vi "WPI_SonarSRF04DigitalOpen.vi"(8 "error in (no error)":errorcluster, 9 "Echo DIO Channel":T1=enum."DIO 2", 11 "Ping DIO Channel":T1=enum."DIO 1") -> (0 "error out":errorcluster, 3 "UltrasonicDevRef":T2={"DevStatus"={"status"=FALSE, "code"=0, "source"=""}, "Ping Channel"=enum."Invalid", "Echo Channel"=enum."Invalid", "CntIndex"=enum."Invalid"})   [LabVIEW 2017]
doc: "Creates a reference to the ultrasonic sensor you specify. You must open a reference before using any other VIs on this palette.\n\nThis software is licensed. Open the labview\\readme\\WPI Robotics Library Open Source License.txt file for more information."
uses:
  <vilib>/Rock Robotics/WPI/Ultrasonic/WPI_UltrasonicDeviceRef.ctl
  <vilib>/Rock Robotics/SystemInterfaces/DIO/FPGA_DIOChannel.ctl
  <vilib>/Rock Robotics/SystemInterfaces/Counter/FPGA_CounterCtrSystemIndex.ctl
  <vilib>/robotics/Simulator/Engine/ctl/DeviceID.ctl
  <vilib>/Rock Robotics/WPI/Counter/WPI_CounterDigitalInputToDigitalSource.vi
  <vilib>/Rock Robotics/WPI/Counter/WPI_CounterOpen Semi Period Mode.vi
  <instrlib>/Devantech SRF05/HAIOL/Simulator/Devantech SRF05 Simulator.lvclass
  <vilib>/robotics/Simulator/NI_Robotics_Simulator.lvlib
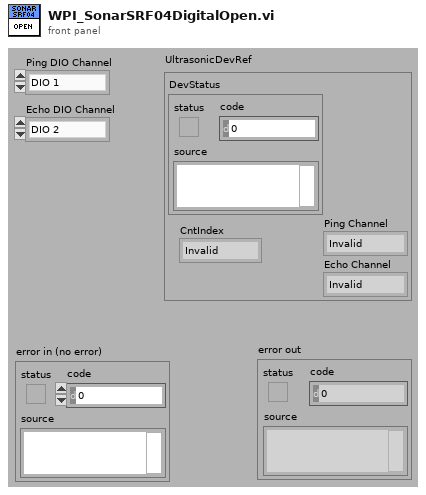
[diagram p1: front panel]
types:
  T1 = typedef "FPGA_DIOChannel.ctl" = enum8{"DIO 0", "DIO 1", "DIO 2", "DIO 3", "DIO 4", "DIO 5", "DIO 6", "DIO 7", "DIO 8", "DIO 9", "DIO MXP 0", "DIO MXP 1", "DIO MXP 2", "DIO MXP 3", "DIO MXP 4", "DIO MXP 5", "DIO MXP 6", "DIO MXP 7", "DIO MXP 8", "DIO MXP 9", "DIO MXP 10", "DIO MXP 11", "DIO MXP 12", "DIO MXP 13", "DIO MXP 14", "DIO MXP 15", "SPI Port CS1", "SPI Port CS2", "SPI Port CS3", "SPI Port MISO", "SPI Port MOSI", "Invalid"}
  T2 = typedef "WPI_UltrasonicDeviceRef.ctl" = cluster{"DevStatus":errorcluster, "Ping Channel":T1, "Echo Channel":T1, "CntIndex":T3}
  T3 = typedef "FPGA_CounterCtrSystemIndex.ctl" = enum8{"Ctr 0", "Ctr 1", "Ctr 2", "Ctr 3", "Ctr 4", "Ctr 5", "Ctr 6", "Ctr 7", "Invalid"}
  T4 = typedef "NI_Robotics_Simulator.lvlib/DeviceID.ctl" = cluster{"robot ID":string, "sensor/actuator ID":string}
  T5 = typedef "WPI_DigitalInputDevRef.ctl" = cluster{"DevStatus":errorcluster, "DIO Channel":T1}
  T6 = typedef "FPGA_CounterEncoderSourceConvertionLVSourceType.ctl" = cluster{"DevStatus":errorcluster, "AnalogTriggerMode?":bool, "DigitalMode":cluster{"DIO Channel":T7}, "AnalogTriggerMode":cluster{"AnalogTriggerIndex":T8, "OutputType":T9}}
  T7 = typedef "FPGA_DIODigitalSourceChannel.ctl" = enum8{"DIO 0", "DIO 1", "DIO 2", "DIO 3", "DIO 4", "DIO 5", "DIO 6", "DIO 7", "DIO 8", "DIO 9", "DIO MXP 0", "DIO MXP 1", "DIO MXP 2", "DIO MXP 3", "DIO MXP 4", "DIO MXP 5", "DIO MXP 6", "DIO MXP 7", "DIO MXP 8", "DIO MXP 9", "DIO MXP 10", "DIO MXP 11", "DIO MXP 12", "DIO MXP 13", "DIO MXP 14", "DIO MXP 15", "Disabled"}
  T8 = typedef "FPGA_AnalogTriggerIndex.ctl" = enum8{"Trig 0", "Trig 1", "Trig 2", "Trig 3", "Trig 4", "Trig 5", "Trig 6", "Trig 7", "Invalid"}
  T9 = typedef "FPGA_AnalogTriggerOutType.ctl" = enum16{"InWindow", "TriggerState", "Rising", "Falling"}
  T10 = typedef "WPI_CounterDevRef.ctl" = cluster{"DevStatus":errorcluster, "CntIndex":T3}
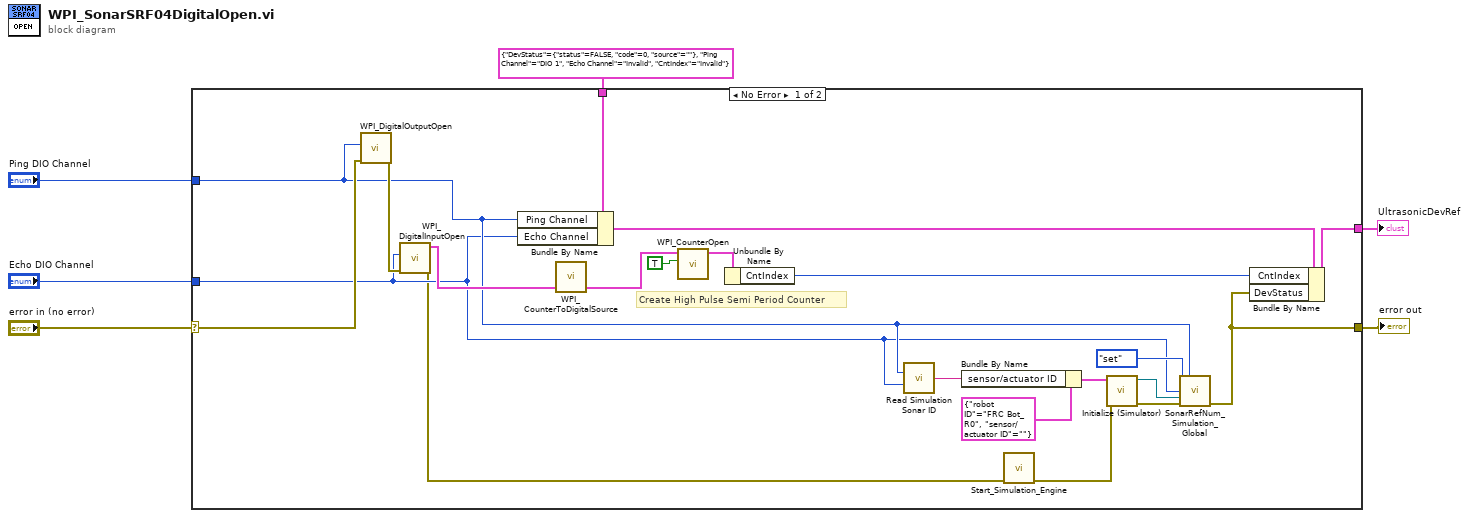
[diagram p0: block diagram]
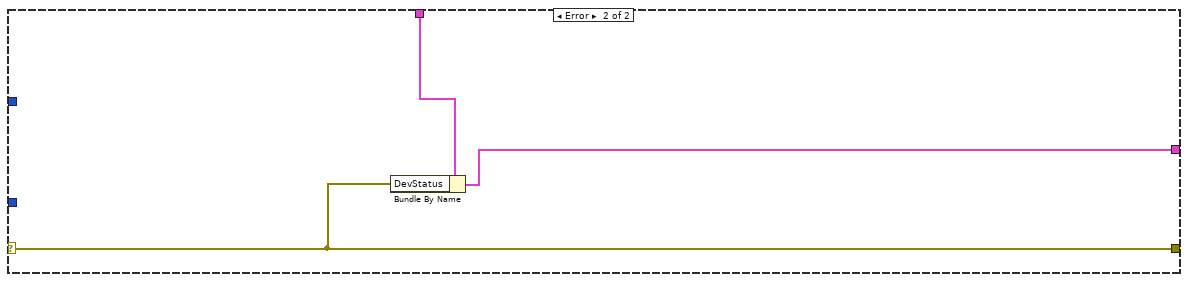
[diagram p2: hidden frame]
diagram:
  n1 = case shown="No Error" "error in (no error)" {
    selector: "error in (no error)" -> [w20 w30]
    tunnel: "Ping DIO Channel" -> [w15 _]
    tunnel: "Echo DIO Channel" -> [w14 _]
    tunnel: [w9 w28] -> w3
    tunnel: [w11 w30] -> w2
    tunnel: T2 {"DevStatus"={"status"=FALSE, "code"=0, "source"=""}, "Ping Channel"=enum."DIO 1", "Echo Channel"=enum."Invalid", "CntIndex"=enum."Invalid"} ("UltrasonicDevRef") -> [w27 w29]
    frame No Error {
      # "Create High Pulse Semi Period Counter"
      n2 = call <vilib>:"WPI_DigitalOutputOpen.vi"("error in (no error)"=w20, "DIO Channel"=w15) -> ("error out"=w25:errorcluster)  [unwired: 1 in, 8 out]
      n3 = call <vilib>:"WPI_DigitalInputOpen.vi"("error in (no error)"=w25, "DIO Channel"=w14) -> ("error out"=w10:errorcluster, "DigitalInputDevRef"=w24:T5)  [unwired: 1 in, 7 out]
      n4 = Bundle By Name(cluster=w27, "Ping Channel"=w15, "Echo Channel"=w14) -> (w21:T2)
      n5 = call-poly <vilib>:"WPI_CounterToDigitalSource.vi"("DigitalInputDevRef"=w24) -> ("Digital Source"=w23:T6)  [unwired: 6 out]
      n6 = call-poly <vilib>:"WPI_CounterOpen.vi"("High Pulse (T)"=TRUE ("High Pulse ? (t)"), "Source"=w23) -> ("CounterDevRef"=w19:T10)  [unwired: 1 in, 8 out]
      n7 = Unbundle By Name(w19) -> ("CntIndex"=w22:T3)
      n8 = call <vilib>:"Read Simulation Sonar ID.vi"("Ping DIO Channel"=w15, "Echo DIO Channel"=w14) -> ("sonar ID"=w18:string)  [unwired: 12 in, 1 out]
      n9 = Bundle By Name(cluster=T4 {"robot ID"="FRC Bot_R0", "sensor/actuator ID"=""} ("Device ID"), "sensor/actuator ID"=w18) -> (w7:T4)
      n10 = call <vilib>:"Start_Simulation_Engine.vi"("error in"=w10) -> ("error out"=w17:errorcluster)  [unwired: 14 in]
      n11 = call <instrlib>:"Initialize (Simulator).vi"("error in (no error)"=w17, "Device ID"=w7) -> ("error out"=w13:errorcluster, "Devantech SRF05 out"=w12:refnum<class "Devantech SRF05.lvclass">)  [unwired: 8 in]
      n12 = call <vilib>:"SonarRefNum_Simulation_Global.vi"("menu"=enum16{"set", "get", "delete"}."set", "Ping DIO Channel"=w15, "Echo DIO Channel"=w14, "Devantech SRF05 Set"=w12, "error in (no error)"=w13) -> ("error out"=w11:errorcluster)  [unwired: 9 in, 1 out]
      n13 = Bundle By Name(cluster=w21, "CntIndex"=w22, "DevStatus"=w11) -> (w9:T2)
    }
    frame Error {
      n14 = Bundle By Name(cluster=w29, "DevStatus"=w30) -> (w28:T2)
    }
  }
  "UltrasonicDevRef" <- w3
  "error out" <- w2
